vi "Filter VIs belonging to Test Case.vi"(8 "error in (no error)":errorcluster, 11 "Array in":path[](array[path])) -> (0 "error out":errorcluster, 3 "Array out":path[](array[path]))   [LabVIEW 2020, in "Coverage Analyzer.lvclass"]
uses:
  Coverage Analyzer.lvclass
  Test Case/LUnit Test Case.lvclass
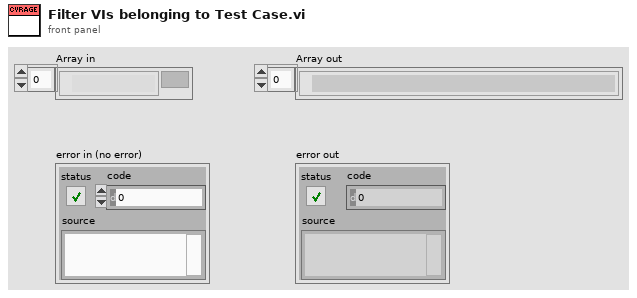
[diagram p1: front panel]
types:
  T1 = typedef "NI.Parent Library Information.ctl" = cluster{"qualified name":string, "localized name":string, "path":path, "parent library kind":T2}
  T2 = typedef "NI.Parent Library Kind.ctl" = enum32{"unknown", "class", "interface"}
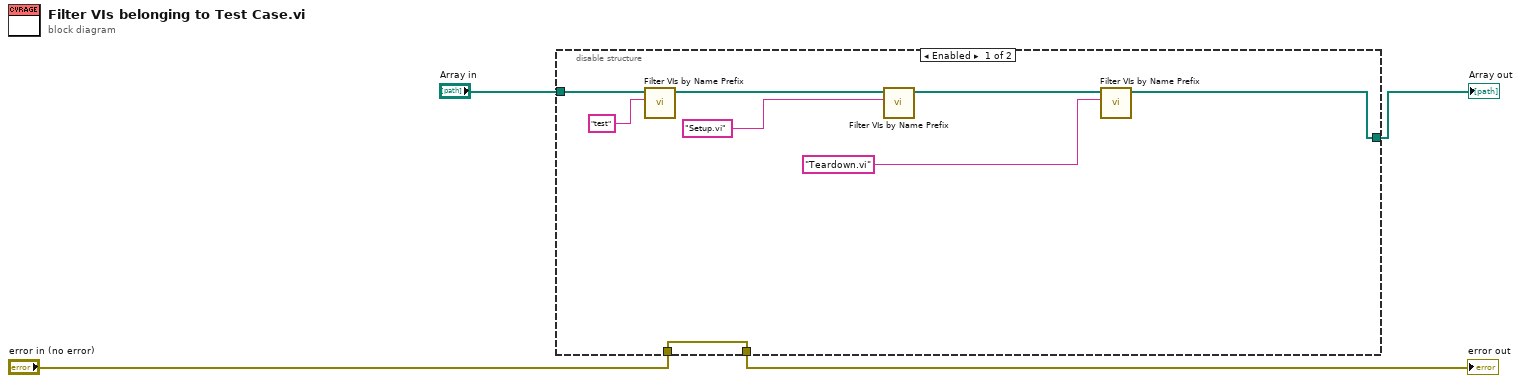
[diagram p0: block diagram]
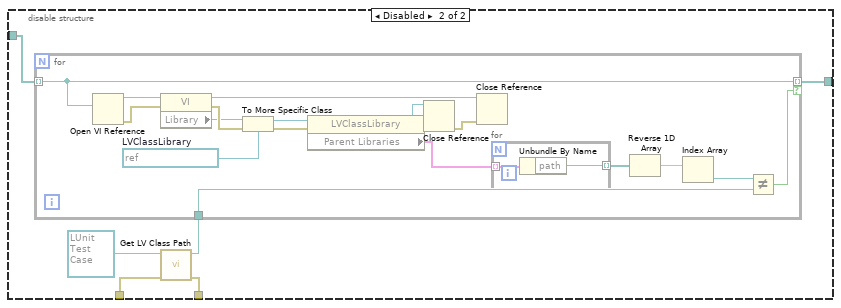
[diagram p2: hidden frame]
diagram:
  n1 = disable-structure shown="Enabled" {
    disable-tunnel: "Array in" -> [w12 w18]
    disable-tunnel: "error in (no error)" -> [w6 w16]
    disable-tunnel: [w6 w15] -> w4
    disable-tunnel: [w5 w13] -> w2
    frame Enabled {
      n2 = call "Filter VIs by Name Prefix.vi"("regular expression"="test", "Array in"=w12) -> ("Array out"=w10:path[])  [unwired: 9 in]
      n3 = call "Filter VIs by Name Prefix.vi"("regular expression"="Setup.vi", "Array in"=w10) -> ("Array out"=w9:path[])  [unwired: 9 in]
      n4 = call "Filter VIs by Name Prefix.vi"("regular expression"="Teardown.vi", "Array in"=w9) -> ("Array out"=w5:path[])  [unwired: 9 in]
    }
    frame Disabled {
      n5 = call <vilib>:"Get LV Class Path.vi"("error in (no error)"=w16, "object"=refnum<class "LUnit Test Case.lvclass"> refnum ("LUnit Test Case.lvclass")) -> ("error out"=w15:errorcluster, "class path"=w14:path)  [unwired: 8 in]
      n6 = for {
        tunnel: w18 -> [w26] mode=indexing
        tunnel: w14 -> [w27]
        tunnel: [w26] -> w13 mode=indexing if=w25
        w21 = refnum<vi> refnum  # LVClassLibrary
        n7 = Open VI Reference(vi path=w26) -> (vi reference=w36:refnum<vi>, error out=w35:errorcluster)  [unwired: 5 in]
        n8 = property class="VI"(reference=w36, error in=w35) -> (reference out=w33:refnum<vi>, error out=w34:errorcluster, "Library"=w23:refnum<vi>)
        n9 = To More Specific Class(target class=w21, reference=w23, error in=w34) -> (specific class reference=w22:refnum<vi>, error out=w24:errorcluster)
        n10 = property class="LVClassLibrary"(reference=w22, error in=w24) -> (reference out=w32:refnum<vi>, error out=w31:errorcluster, "Parent Libraries"=w20:T1[])
        n11 = Close Reference(reference=w32, error in (no error)=w31) -> (error out=w30:errorcluster)
        n12 = Close Reference(reference=w33, error in (no error)=w30) -> ()  [unwired: 1 out]
        n13 = for {
          tunnel: w20 -> [w38] mode=indexing
          tunnel: [w37] -> w19 mode=indexing
          n14 = Unbundle By Name(w38) -> ("path"=w37:path)
        }
        n15 = Reverse 1D Array(array=w19) -> (reversed array=w29:path[])
        n16 = Index Array(array=w29) -> (element=w28:path)  [unwired: 1 in]
        n17 = Not Equal?(x=w28, y=w27) -> (x != y?=w25:bool)
      }
    }
  }
  "error out" <- w4
  "Array out" <- w2
